vi "Lvi Clock Settings.vi"(0 "TaskRef":i32, 1 "SetFrequency":bool, 2 "SetSource":bool, 5 "ClockFrequency":dbl, 7 "ExternalDivider":u32, 9 "InternalSource":bool, 11 "error in (no error)":errorcluster, 12 "SetDivider":bool) -> (3 "function return":u32(ring), 4 "TaskRef out":i32, 6 "ClockFrequency out":dbl, 8 "ExternalDivider out":u32, 10 "InternalSource out":bool, 15 "error out":errorcluster)   [LabVIEW 2022 SP3, in "DtLvLink.lvlib"]
doc: "Calls directly into the entry points of the DLL of the Data Acq SDK to set clock properties and return information about the clock properties of the device. This VI is used by the higher-level VI, DtOLClock."
uses:
  DtLvLink.lvlib
  <userlib>/LV-Link3/DtLvLink_64.dll
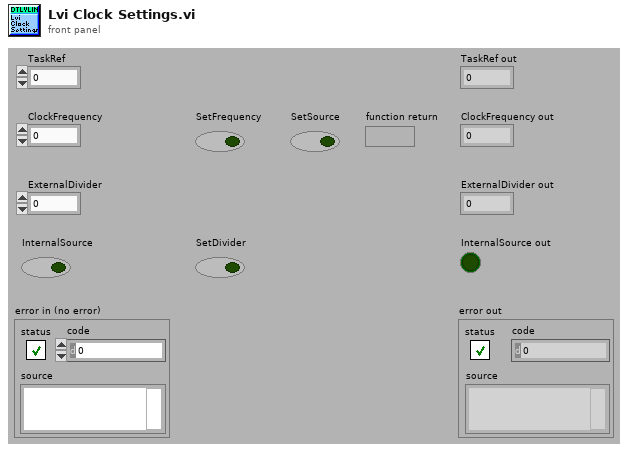
[diagram p1: front panel]
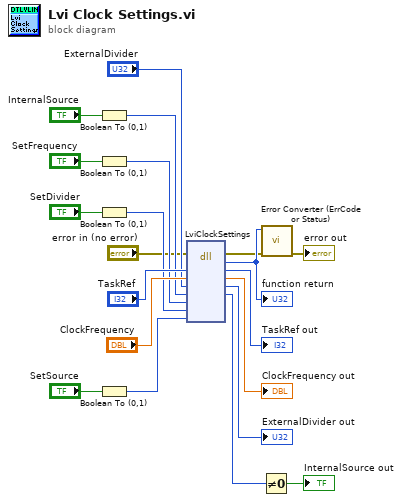
[diagram p0: block diagram]
diagram:
  n1 = Boolean To (0,1)(Boolean="InternalSource") -> (0, 1=w12:i16)
  n2 = Boolean To (0,1)(Boolean="SetFrequency") -> (0, 1=w8:i16)
  n3 = Boolean To (0,1)(Boolean="SetDivider") -> (0, 1=w6:i16)
  n4 = Boolean To (0,1)(Boolean="SetSource") -> (0, 1=w4:i16)
  n5 = dll-call lib="C:/Program Files/National Instruments/LabVIEW 2022/user.lib/LV-Link3/DtLvLink_64.*" fn="LviClockSettings"(error in="error in (no error)", "TaskRef"="TaskRef", "ClockFrequency"="ClockFrequency", "ExternalDivider"="ExternalDivider", "InternalSource"=w12, "SetFrequency"=w8, "SetDivider"=w6, "SetSource"=w4) -> (error out=w2:errorcluster, w20:u32, "TaskRef"=→"TaskRef out":i32, "ClockFrequency"=→"ClockFrequency out":dbl, "ExternalDivider"=→"ExternalDivider out":u32, "InternalSource"=w10:u8)  [unwired: 5 in, 1 out]
  "function return" <- w20
  n6 = Not Equal To 0?(x=w10) -> (x != 0?=→"InternalSource out":bool)
  n7 = call "Error Converter (ErrCode or Status).vi"("error in (no error)"=w2, "error code"=w20) -> ("error out"=→"error out":errorcluster)  [unwired: 9 in]
